vi "_emi_Version Holder.vi"(1 "Action(GET)":enum16{"GET", "SET"}(ring), 7 "Version Info in":T1={"Name"="Default Name", "Major"=0, "Minor"=0, "Fix"=0, "Build"=0, "Type"=enum."Alfa", "Dev"=FALSE, "Version Name"="", "Date"=timestamp(0 s since 1904-01-01)} {"Date" format="%<%y%m%d>T"}, 11 "error in (no error)":errorcluster) -> (4 "Version set":bool, 8 "Version Info out":T1={"Name"="Default Name", "Major"=0, "Minor"=0, "Fix"=0, "Build"=0, "Type"=enum."Alfa", "Dev"=FALSE, "Version Name"="", "Date"=timestamp(0 s since 1904-01-01)} {"Date" format="%<%y%m%d>T"}, 15 "error out":errorcluster)   [LabVIEW 2011]
uses:
  emi_Version Info.ctl
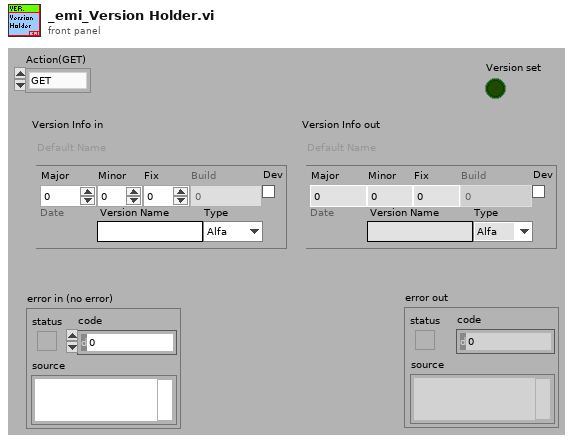
[diagram p1: front panel]
types:
  T1 = typedef "emi_Version Info.ctl" = cluster{"Name":string, "Major":i16, "Minor":i16, "Fix":i16, "Build":i32, "Type":enum16{"Alfa", "Beta", "Stable"}, "Dev":bool, "Version Name":string, "Date":timestamp}
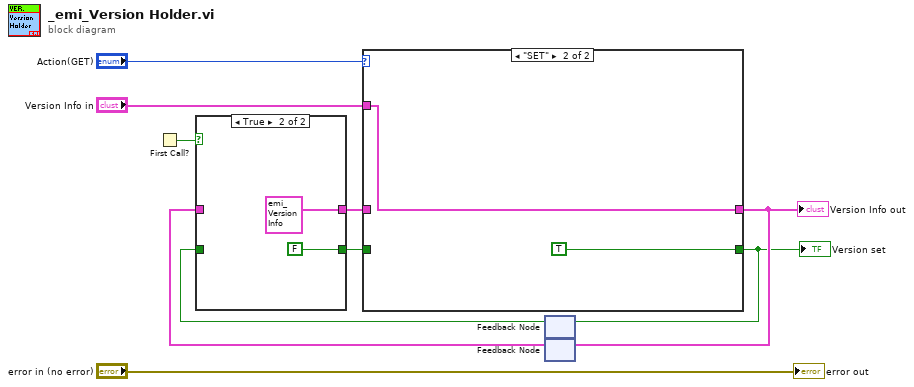
[diagram p0: block diagram]
diagram:
  n1 = First Call?() -> (First Call?: T/F=w7:bool)
  n2 = feedback #1() -> (w1:bool)  [unwired: 1 in]
  n3 = feedback #2() -> (w8:T1)  [unwired: 1 in]
  n4 = case shown="True" w7 {
    tunnel: w8 -> [w12 _]
    tunnel: [w12 T1 {"Name"="Default Name", "Major"=0, "Minor"=0, "Fix"=0, "Build"=0, "Type"=enum."Alfa", "Dev"=FALSE, "Version Name"="", "Date"=timestamp(0 s since 1904-01-01)} ("Version Info")] -> w5
    tunnel: [w11 FALSE] -> w3
    tunnel: w1 -> [w11 _]
    frame False {
    }
    frame True {
    }
  }
  n5 = case shown="\"SET\"" "Action(GET)" {
    tunnel: [w16 w18] -> w6
    tunnel: w5 -> [w16 _]
    tunnel: "Version Info in" -> [_ w18]
    tunnel: [w15 TRUE] -> w2
    tunnel: w3 -> [w15 _]
    frame "GET", Default {
    }
    frame "SET" {
    }
  }
  "Version Info out" <- w6
  "Version set" <- w2
  n6 = feedback-in #1(w2) -> ()
  n7 = feedback-in #2(w6) -> ()
  "error out" <- "error in (no error)"
